vi "Test Deserialize Variable Sized Arrays.vi"(8 "error in (no error)":errorcluster) -> (0 "error out":errorcluster)   [LabVIEW 2013]
uses:
  src/JKI JSON Serialization.lvlib
  <vilib>/addons/_JKI Toolkits/Caraya/classes/Test/Test.lvclass
  <vilib>/addons/_JKI Toolkits/Caraya/classes/Assert/Assert.lvclass
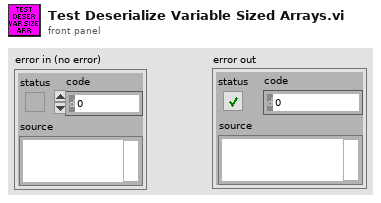
[diagram p1: front panel]
types:
  T1 = cluster{"hello":string, "wolrd":string, "values":string[][]}
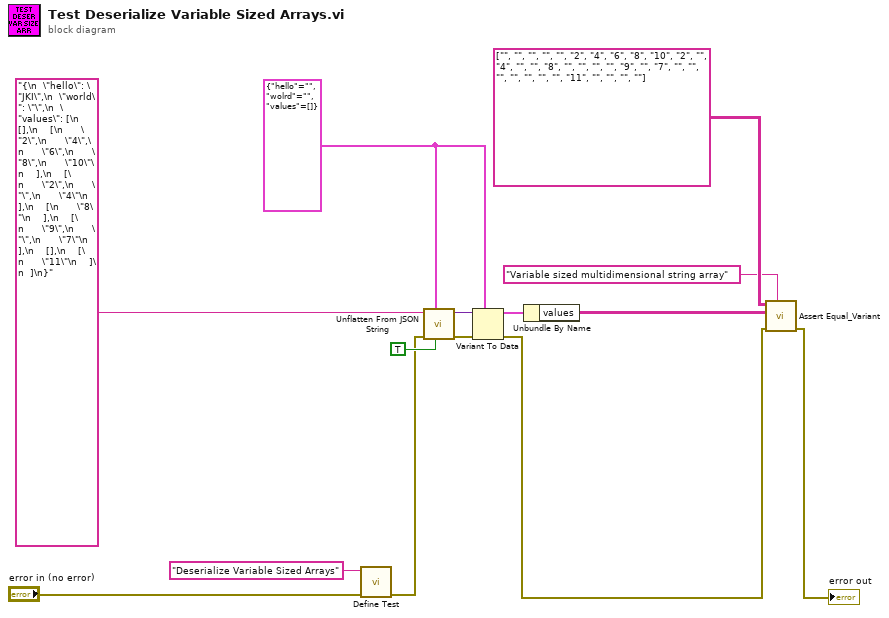
[diagram p0: block diagram]
diagram:
  w13 = T1 {"hello"="", "wolrd"="", "values"=[]}
  n1 = call <vilib>:"Define Test.vi"("error in (no error)"="error in (no error)", "Label (VI Title)"="Deserialize Variable Sized Arrays") -> ("error out"=w7:errorcluster)  [unwired: 9 in]
  n2 = call "Unflatten From JSON String.vi"("Nulls as Defaults (T)"=TRUE, "Type and Defaults"=w13, "error in (no error)"=w7, "JSON String"="{\n  \"hello\": \"JKI\",\n  \"world\": \"\",\n  \"values\": [\n    [],\n    [\n      \"2\",\n      \"4\",\n      \"6\",\n      \"8\",\n      \"10\"\n    ],\n    [\n      \"2\",\n      \"\",\n      \"4\"\n    ],\n    [\n      \"8\"\n    ],\n    [\n      \"9\",\n      \"\",\n      \"7\"\n    ],\n    [],\n    [\n      \"11\"\n    ]\n  ]\n}") -> ("error out"=w12:errorcluster, "Variant"=w11:variant)  [unwired: 6 in]
  n3 = Variant To Data(error in=w12, type=w13, Variant=w11) -> (data=w8:T1, error out=w3:errorcluster)
  n4 = Unbundle By Name(w8) -> ("values"=w5:string[][])
  n5 = call <vilib>:"Assert Equal_Variant.vi"("Label"="Variable sized multidimensional string array", "error in (no error)"=w3, "Y"=w5, "X"=string[][] [["", "", "", "", ""], ["2", "4", "6", "8", "10"], ["2", "", "4", "", ""], ["8", "", "", "", ""], ["9", "", "7", "", ""], ["", "", "", "", ""], ["11", "", "", "", ""]]) -> ("error out"=→"error out":errorcluster)  [unwired: 7 in]
